vi "add and substract.vi"() -> ()   [LabVIEW 2016]
panel:
  in  "stop":bool
  out "N1-N2":dbl
  out "N1+N2":dbl
  in  "Number2":dbl
  in  "Number1":dbl
  # "Add and Subtract"
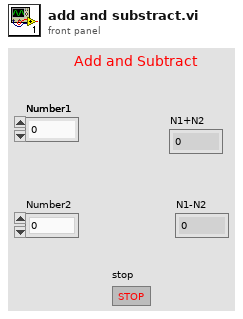
[diagram p1: front panel]
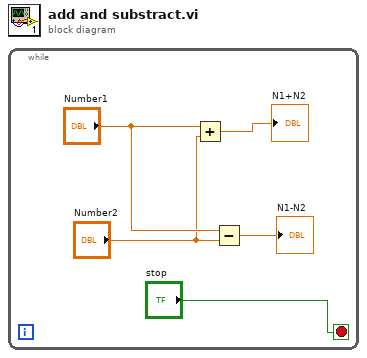
[diagram p0: block diagram]
diagram:
  n1 = while {
    stop <- "stop" stop-if-true
    n2 = Add(x="Number1", y="Number2") -> (x+y=→"N1+N2":dbl)
    n3 = Subtract(x="Number1", y="Number2") -> (x-y=→"N1-N2":dbl)
  }
